vi "setUp.vi"(8 "error in":errorcluster, 11 "reference in":refnum<class "Single Core Acyclic Loopback.lvclass">) -> (0 "error out":errorcluster, 3 "reference out":refnum<class "Single Core Acyclic Loopback.lvclass">)   [LabVIEW 2020, in "Single Core Acyclic Loopback.lvclass"]
doc: "setUp runs prior to the test method during test execution. Use this method to initialize any object data required by your tests."
uses:
  Single Core Acyclic Loopback.lvclass
  C:/Program Files (x86)/National Instruments/LabVIEW 2020/vi.lib/addons/_JKI Toolkits/VI Tester/TestCase.llb/TestCase.lvclass
  <vilib>/addons/_JKI Toolkits/VI Tester/TestCase.llb/TestCase.lvclass
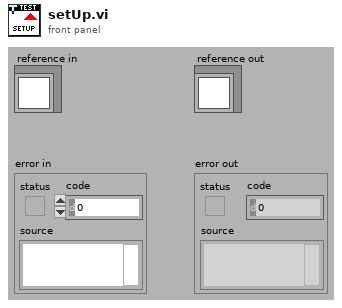
[diagram p1: front panel]
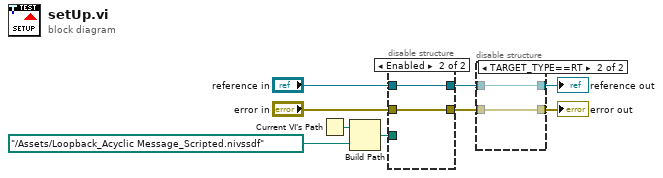
[diagram p0: block diagram]
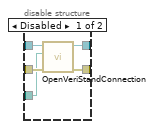
[diagram p2: hidden frame]
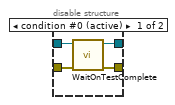
[diagram p3: hidden frame]
diagram:
  n1 = Current VI's Path() -> (path=w3:path)
  n2 = Build Path(base path=w3, name or relative path=path "../Assets/Loopback_Acyclic Message_Scripted.nivssdf" ("Hardware File Path")) -> (appended path=w1:path)
  n3 = disable-structure shown="Enabled" {
    disable-tunnel: "reference in" -> [w14 w16]
    disable-tunnel: [w13 w16] -> w6
    disable-tunnel: "error in" -> [w12 w15]
    disable-tunnel: [w11 w15] -> w4
    disable-tunnel: w1 -> [w10 _]
    frame Disabled {
      n4 = call-dynamic "OpenVeriStandConnection.vi"("error in (no error)"=w12, "System Definition File"=w10, "VeriStand Test Case in"=w14) -> ("error out"=w11:errorcluster, "VeriStand Test Case out"=w13:refnum<class "Single Core Acyclic Loopback.lvclass">)  [unwired: 6 in, 1 out]
    }
    frame Enabled {
    }
  }
  n5 = disable-structure shown="TARGET_TYPE==RT" {
    disable-tunnel: w4 -> [w20 w21]
    disable-tunnel: [w19 w21] -> w9
    disable-tunnel: [w18 w22] -> w8
    disable-tunnel: w6 -> [w17 w22]
    frame condition #0 (active) {
      n6 = call <vilib>:"WaitOnTestComplete.vi"("error in (no error)"=w20, "TestCase in"=w17) -> ("error out"=w19:errorcluster, "TestCase out"=w18:refnum<class "Single Core Acyclic Loopback.lvclass">)  [unwired: 8 in]
    }
    frame condition #1 {
    }
  }
  "error out" <- w9
  "reference out" <- w8
